vi "Convert Fahrenheit to Celsius.vi"(1 "Fahrenheit":dbl, 2 "Boolean":bool) -> (0 "Celsius":dbl)   [LabVIEW 2021]
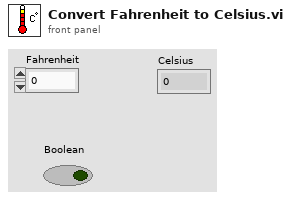
[diagram p1: front panel]
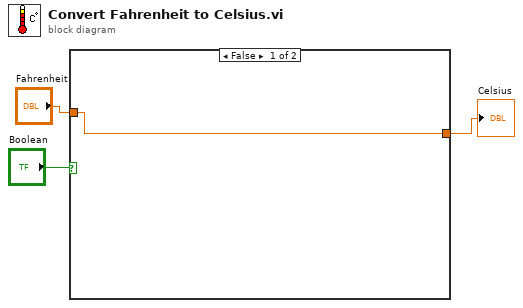
[diagram p0: block diagram]
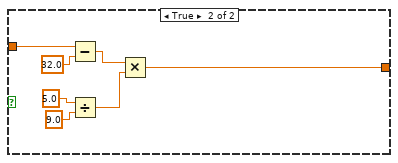
[diagram p2: hidden frame]
diagram:
  n1 = case shown="False" "Boolean" {
    tunnel: "Fahrenheit" -> [w4 w9]
    tunnel: [w4 w5] -> w1
    frame False {
    }
    frame True {
      n2 = Subtract(x=w9, y=32.0) -> (x-y=w7:dbl)
      n3 = Divide(x=5.0, y=9.0) -> (x/y=w6:dbl)
      n4 = Multiply(x=w7, y=w6) -> (x*y=w5:dbl)
    }
  }
  "Celsius" <- w1
